vi "Receive.vi"(11 "Queue Transport in":refnum<class "Queue Transport.lvclass">) -> (0 "Error out":errorcluster, 2 "Msg":refnum<class "Msg.lvclass">)   [LabVIEW 2025, in "jettl.lvlib" / "Transport.lvlib" / "Queue Transport.lvclass"]
uses:
  Queue Transport.lvclass
  Queue Transport.lvclass/Queue Transport.ctl
  Msg/Msg.lvclass
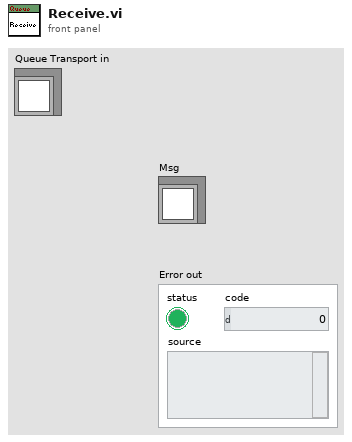
[diagram p1: front panel]
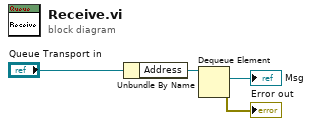
[diagram p0: block diagram]
diagram:
  n1 = Unbundle By Name("Queue Transport in") -> ("Address"=w3:refnum<queue>)
  n2 = Dequeue Element(queue=w3) -> (element=→"Msg":refnum<class "Msg.lvclass">, error out=→"Error out":errorcluster)  [unwired: 2 in, 2 out]
